vi "Read ProjectItem idx.vi"(11 "BuildManager in":refnum<class "BuildManager.lvclass">) -> (2 "ProjectItem idx":i32=-1, 3 "BuildManager out":refnum<class "BuildManager.lvclass">)   [LabVIEW 2020, in "SolutionBuilder.lvlib" / "BuildManager.lvclass"]
uses:
  BuildManager.lvclass
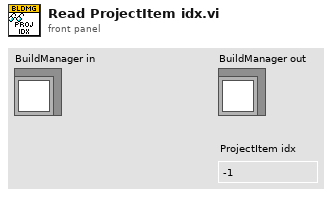
[diagram p1: front panel]
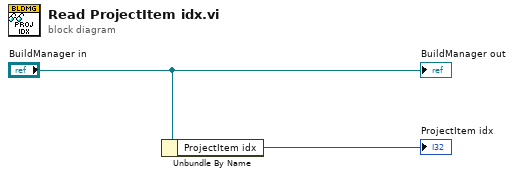
[diagram p0: block diagram]
diagram:
  n1 = Unbundle By Name("BuildManager in") -> ("ProjectItem idx"=→"ProjectItem idx":i32)
  "BuildManager out" <- "BuildManager in"
